vi "convertADCsToVolts.vi"(8 "error in (no error)":errorcluster, 11 "ILC in":refnum<class "ILC.lvclass">) -> (0 "error out":errorcluster, 3 "ILC out":refnum<class "ILC.lvclass">)   [LabVIEW 2015, in "ILCCommon.lvlib" / "ILC.lvclass"]
uses:
  <userlib>/Common/ILC/ILC/ILC.lvclass
  <userlib>/Common/ILC/ILC/ILC.lvclass/ILC.ctl
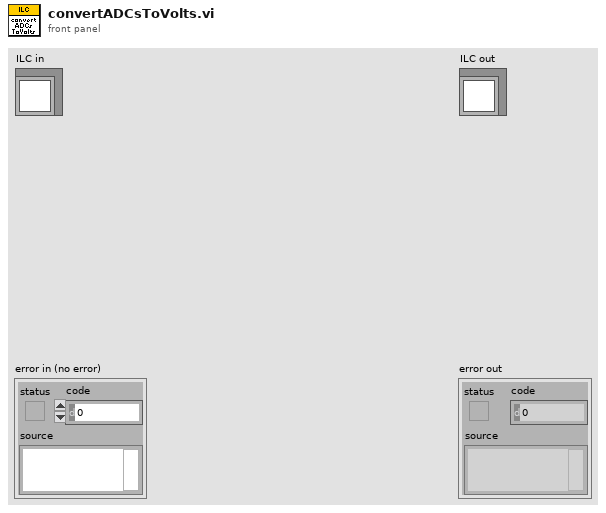
[diagram p1: front panel]
types:
  T1 = typedef "ILCCommon.lvlib/ILCConfiguration.lvlib/ADC Conversion Settings.ctl" = cluster{"Reference Voltage Vref":dbl[unit], "Nominal Input Range in Counts":u32, "Preamplifier Gain (K1 * K2)":dbl, "Conversion Settling Cycles":u16, "Excitation Voltage Vexc":dbl[unit]}
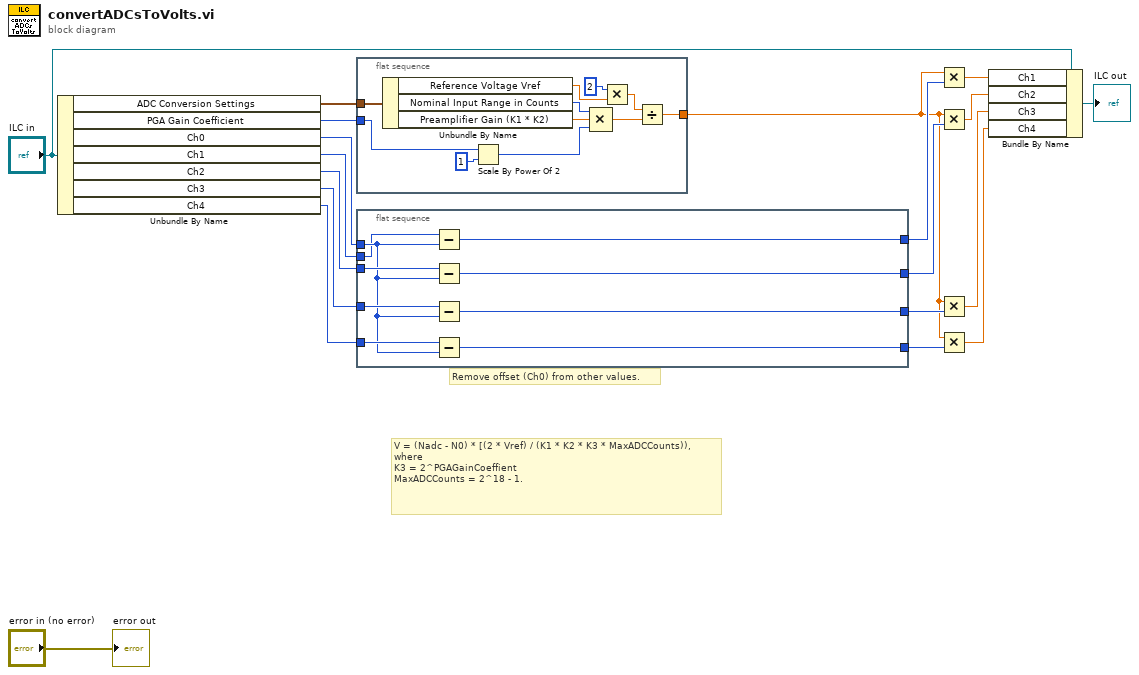
[diagram p0: block diagram]
diagram:
  # "V = (Nadc - N0) * [(2 * Vref) / (K1 * K2 * K3 * MaxADCCounts)),\nwhere\nK3 = 2^PGAGainCoeffient\nMaxADCCounts = 2^18 - 1."
  # "Remove offset (Ch0) from other values."
  n1 = Unbundle By Name("ILC in") -> ("ADC Conversion Settings"=w2:T1, "PGA Gain Coefficient"=w1:u8, "Ch0"=w12:i32, "Ch1"=w16:i32, "Ch2"=w15:i32, "Ch3"=w14:i32, "Ch4"=w13:i32)
  n2 = flat-sequence {
    tunnel: [w26] -> w8
    tunnel: w2 -> [w24]
    tunnel: w1 -> [w23]
    frame #0 {
      n3 = Unbundle By Name(w24) -> ("Reference Voltage Vref"=w21:dbl[unit], "Nominal Input Range in Counts"=w30:u32, "Preamplifier Gain (K1 * K2)"=w29:dbl)
      n4 = Scale By Power Of 2(n=w23, x=u8 1) -> (x*2^n=w28:u8)
      n5 = Compound Arithmetic op=MULTIPLY(w30, w29, w28) -> (w27:dbl)
      n6 = Multiply(x=2, y=w21) -> (x*y=w20:dbl[unit])
      n7 = Divide(x=w20, y=w27) -> (x/y=w26:dbl[unit])
    }
  }
  n8 = flat-sequence {
    tunnel: w16 -> [w31]
    tunnel: w15 -> [w39]
    tunnel: w14 -> [w38]
    tunnel: w13 -> [w37]
    tunnel: w12 -> [w36]
    tunnel: [w35] -> w11
    tunnel: [w34] -> w10
    tunnel: [w33] -> w9
    tunnel: [w32] -> w7
    frame #0 {
      n9 = Subtract(x=w31, y=w36) -> (x-y=w35:i32)
      n10 = Subtract(x=w39, y=w36) -> (x-y=w34:i32)
      n11 = Subtract(x=w38, y=w36) -> (x-y=w33:i32)
      n12 = Subtract(x=w37, y=w36) -> (x-y=w32:i32)
    }
  }
  n13 = Multiply(x=w8, y=w11) -> (x*y=w6:dbl[unit])
  n14 = Multiply(x=w8, y=w10) -> (x*y=w5:dbl[unit])
  n15 = Multiply(x=w8, y=w9) -> (x*y=w4:dbl[unit])
  n16 = Multiply(x=w8, y=w7) -> (x*y=w3:dbl[unit])
  n17 = Bundle By Name(cluster="ILC in", "Ch1"=w6, "Ch2"=w5, "Ch3"=w4, "Ch4"=w3) -> (→"ILC out":refnum<class "ILC.lvclass">)
  "error out" <- "error in (no error)"
